vi "Data_processing.vi"(4 "Presssure":T2 {"Pressure (barg)" scale=0.0..70.0}, 5 "Auxiliary":T3 {"Absolute adsorption" items=["Micropore_filling", "Surface_coverage"]; "EOS" items=["Ideal", "CH4_van_der_Waal", "CH4_Redlich_Kwong", "CO2_van_der_Waal", "CO2_Redlich_Kwong", ""]}) -> (0 "z":dbl, 1 "Latest Data":T1 {"Temperature" scale=0.0..100.0; "Pressure (barg)" scale=0.0..70.0}, 3 "rho_bulk":dbl)   [LabVIEW 2016]
uses:
  auxiliary_cluster.ctl
  EOS.ctl
  pressure_cluster.ctl
  adsorbed_cluster.ctl
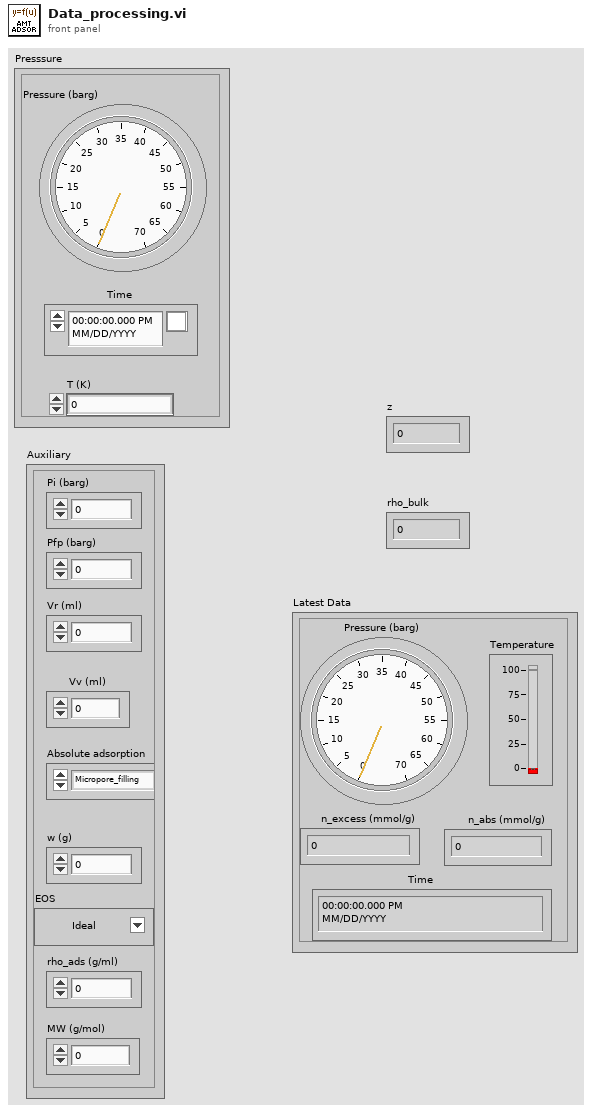
[diagram p1: front panel]
types:
  T1 = typedef "adsorbed_cluster.ctl" = cluster{"Time":timestamp, "Pressure (barg)":dbl, "n_excess (mmol/g)":dbl, "n_abs (mmol/g)":dbl, "Temperature":dbl}
  T2 = typedef "pressure_cluster.ctl" = cluster{"Time":timestamp, "Pressure (barg)":dbl, "T (K)":dbl}
  T3 = typedef "auxiliary_cluster.ctl" = cluster{"Pi (barg)":dbl, "Pfp (barg)":dbl, "Vr (ml)":dbl, "w (g)":dbl, "EOS":T4, "rho_ads (g/ml)":dbl, "MW (g/mol)":dbl, "Vv (ml)":dbl, "Absolute adsorption":u16}
  T4 = typedef "EOS.ctl" = u16
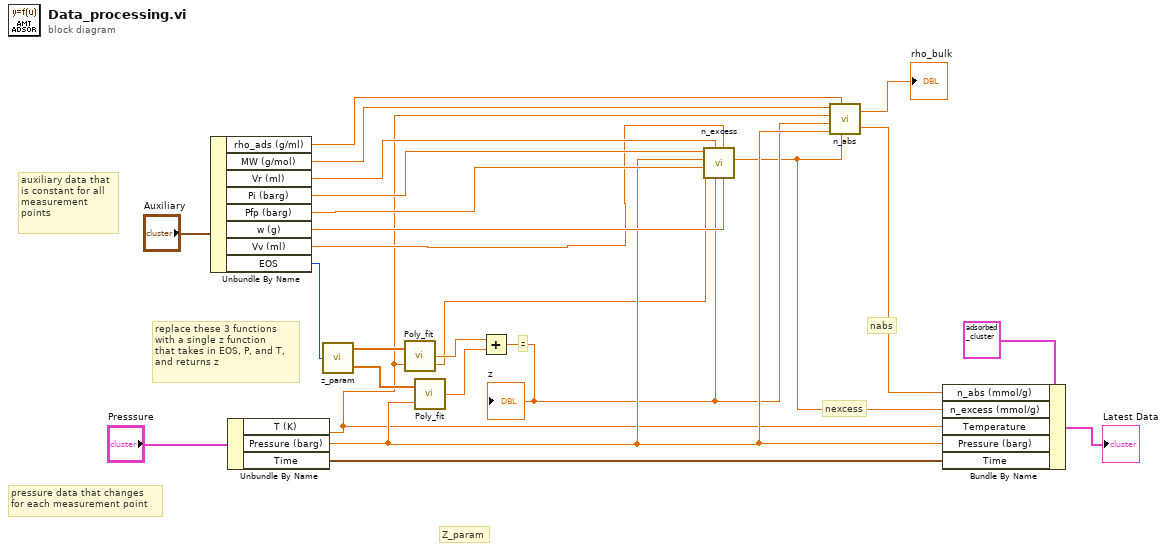
[diagram p0: block diagram]
diagram:
  # "replace these 3 functions\nwith a single z function \nthat takes in EOS, P, and T, \nand returns z"
  # "pressure data that changes\nfor each measurement point"
  # "auxiliary data that \nis constant for all\nmeasurement \npoints"
  # "nabs"
  # "nexcess"
  # "Z_param"
  # "z"
  n1 = Unbundle By Name("Auxiliary") -> ("rho_ads (g/ml)"=w7:dbl, "MW (g/mol)"=w8:dbl, "Vr (ml)"=w11:dbl, "Pi (barg)"=w12:dbl, "Pfp (barg)"=w13:dbl, "w (g)"=w14:dbl, "Vv (ml)"=w4:dbl, "EOS"=w5:T4)
  n2 = Unbundle By Name("Presssure") -> ("T (K)"=w1:dbl, "Pressure (barg)"=w10:dbl, "Time"=w21:timestamp)
  n3 = call "z_param.vi"("EOS"=w5) -> ("z_Param_T"=w18:dbl[], "z_Param_P"=w17:dbl[])
  n4 = call "Poly_fit.vi"("Input"=w1, "Parameters"=w18) -> ("Output"=w15:dbl)
  n5 = call "Poly_fit.vi"("Input"=w10, "Parameters"=w17) -> ("Output"=w16:dbl)
  n6 = Add(x=w15, y=w16) -> (x+y=w9:dbl)
  "z" <- w9
  n7 = call "n_excess.vi"("w"=w14, "Vv"=w4, "z"=w9, "Vr"=w11, "T"=w1, "Pfp"=w13, "Pf"=w10, "Pi"=w12) -> ("nexcess"=w2:dbl)  [unwired: 3 in]
  n8 = call "n_abs.vi"("n_excess"=w2, "rho_ads"=w7, "Pf"=w10, "z"=w9, "T"=w1, "MW"=w8) -> ("n_abs"=w3:dbl, "rho_bulk"=→"rho_bulk":dbl)
  n9 = Bundle By Name(cluster=T1 {"Time"=timestamp(0 s since 1904-01-01), "Pressure (barg)"=0.0, "n_excess (mmol/g)"=0.0, "n_abs (mmol/g)"=0.0, "Temperature"=0.0} ("Adsorbed"), "n_abs (mmol/g)"=w3, "n_excess (mmol/g)"=w2, "Temperature"=w1, "Pressure (barg)"=w10, "Time"=w21) -> (→"Latest Data":T1)
